vi "Launch Task Settings.vi"(8 "error in (no error)":errorcluster, 10 "User Selections":i32[](array[numeric]), 11 "BuildServer in":refnum<class "BuildServer.lvclass">) -> (0 "error out":errorcluster, 3 "BuildServer out":refnum<class "BuildServer.lvclass">)   [LabVIEW 2017, in "BuildServer.lvlib" / "BuildServer.lvclass"]
uses:
  BuildServer.lvclass
  <vilib>/ActorFramework/Actor/Actor.lvclass
  Task Setting Editor/Task Setting Editor/Task Setting Editor.lvclass
  Task Setting Editor/Task Setting Editor Messages/Set Task List Msg/Set Task List Msg.lvclass
  Task Setting Editor/Task Setting Editor Messages/Populate Worker Ring Msg/Populate Worker Ring Msg.lvclass
  Task Setting Editor/Task Setting Editor Messages/Open FrontPanel Msg/Open FrontPanel Msg.lvclass
  <vilib>/ActorFramework/Message Enqueuer/Message Enqueuer.lvclass
  <vilib>/ActorFramework/Message/Message.lvclass
  Volumes/Data/Users/benji667/Git/BuildFarm/WebSocket Server/Actors/Actor wHelper/Actor wHelper/Actor wHelper.lvclass
  Volumes/Data/Users/benji667/Git/BuildFarm/WebSocket Server/Actors/Actor wHelper/Actor wLauncher/Actor wLauncher.lvclass
  Volumes/Data/Users/benji667/Git/BuildFarm/WebSocket Server/Actors/Actor wHelper/Actor wUI/Actor wUI.lvclass
  Applications/National Instruments/LabVIEW 2017 64-bit/vi.lib/ActorFramework/Actor/Actor.lvclass
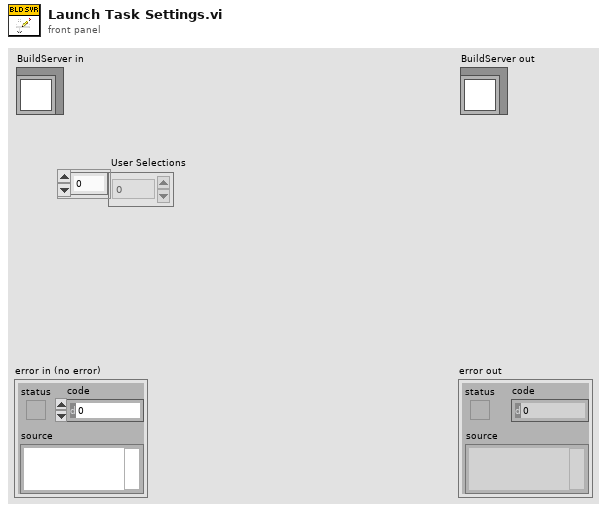
[diagram p1: front panel]
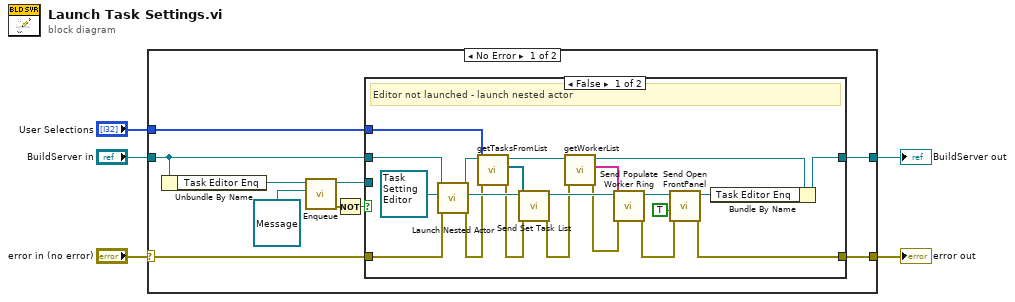
[diagram p0: block diagram]
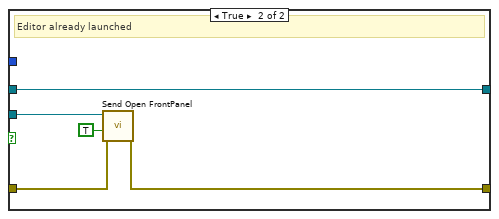
[diagram p2: hidden frame]
diagram:
  n1 = case shown="No Error" "error in (no error)" {
    selector: "error in (no error)" -> [w14 w42]
    tunnel: [w13 w42] -> w4
    tunnel: [w12 w41] -> w2
    tunnel: "BuildServer in" -> [w11 w41]
    tunnel: "User Selections" -> [w15 _]
    frame No Error {
      n2 = Unbundle By Name(w11) -> ("Task Editor Enq"=w10:refnum<class "Message Enqueuer.lvclass">)
      n3 = call <vilib>:"Enqueue.vi"("Message"=refnum<class "Message.lvclass"> refnum, "Message Enqueuer in"=w10) -> ("error out"=w7:errorcluster, "Message Enqueuer out"=w9:refnum<class "Message Enqueuer.lvclass">)  [unwired: 8 in]
      n4 = Not(x=w7) -> (.not. x?=w6:bool)
      n5 = case shown="False" w6 {
        tunnel: w15 -> [w24 _]
        tunnel: w14 -> [w33 w37]
        tunnel: [w26 w36] -> w13
        tunnel: [w30 w40] -> w12
        tunnel: w11 -> [w31 w40]
        tunnel: w9 -> [_ w39]
        frame False {
          # "Editor not launched - launch nested actor"
          n6 = call <vilib>:"Launch Nested Actor.vi"("error in (no error)"=w33, "Nested Actor"=refnum<class "Task Setting Editor.lvclass"> refnum ("Task Setting Editor.lvlib:Task Setting Editor.lvclass"), "Caller Actor in"=w31) -> ("error out"=w23:errorcluster, "Nested Actor's Enqueuer"=w34:refnum<class "Message Enqueuer.lvclass">, "Caller Actor out"=w20:refnum<class "BuildServer.lvclass">)  [unwired: 6 in]
          n7 = call "getTasksFromList.vi"("error in (no error)"=w23, "User Selection"=w24, "BuildServer in"=w20) -> ("error out"=w22:errorcluster, "Selected Tasks"=w21:refnum<class "Task.lvclass">[])  [unwired: 7 in]
          n8 = call "Send Set Task List.vi"("error in (no error)"=w22, "Task List"=w21, "Message Enqueuer"=w34) -> ("error out"=w18:errorcluster, "Message Enqueuer out"=w32:refnum<class "Message Enqueuer.lvclass">)  [unwired: 7 in]
          n9 = call "getWorkerList.vi"("error in (no error)"=w18, "BuildServer in"=w20) -> ("error out"=w17:errorcluster, "Worker List"=w16:string[], "BuildServer out"=w19:refnum<class "BuildServer.lvclass">)  [unwired: 7 in]
          n10 = call "Send Populate Worker Ring.vi"("error in (no error)"=w17, "Worker List"=w16, "Message Enqueuer"=w32) -> ("error out"=w27:errorcluster, "Message Enqueuer out"=w29:refnum<class "Message Enqueuer.lvclass">)  [unwired: 7 in]
          n11 = call "Send Open FrontPanel.vi"("error in (no error)"=w27, "Open"=TRUE, "Message Enqueuer"=w29) -> ("error out"=w26:errorcluster, "Message Enqueuer out"=w28:refnum<class "Message Enqueuer.lvclass">)  [unwired: 7 in]
          n12 = Bundle By Name(cluster=w19, "Task Editor Enq"=w28) -> (w30:refnum<class "BuildServer.lvclass">)
        }
        frame True {
          # "Editor already launched"
          n13 = call "Send Open FrontPanel.vi"("error in (no error)"=w37, "Open"=TRUE, "Message Enqueuer"=w39) -> ("error out"=w36:errorcluster)  [unwired: 7 in, 1 out]
        }
      }
    }
    frame Error {
    }
  }
  "error out" <- w4
  "BuildServer out" <- w2
